vi "Shooter Distance.vi"() -> ()   [LabVIEW 2016]
panel:
  out "S)(0073R D1574NC3":dbl
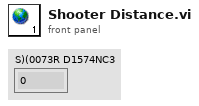
[diagram p1: front panel]
diagram:
